vi "获取队列引用.vi"(8 "错误输入（无错误）":errorcluster) -> (0 "错误输出":errorcluster, 3 "队列组":T1)   [LabVIEW 2020]
uses:
  viLib/QueueLib/QueueLib.lvlib
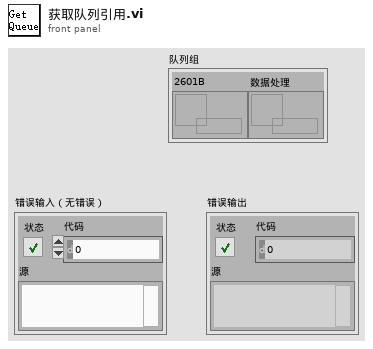
[diagram p1: front panel]
types:
  T1 = typedef "队列组.ctl" = cluster{"2601B":refnum<queue>, "数据处理":refnum<queue>}
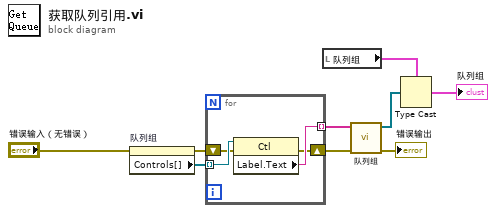
[diagram p0: block diagram]
diagram:
  n1 = property on="队列组" class="Clust (严格)"(error in="错误输入（无错误）") -> (error out=w3:errorcluster, "Controls[]"=w6:refnum<vi>[])  [unwired: 1 in, 1 out]
  n2 = for {
    tunnel: w6 -> [w13] mode=indexing
    tunnel: [w12] -> w5 mode=indexing
    shift-right: [w10] -> w2
    shift-left: w3 -> [w11]
    n3 = property class="Ctl"(reference=w13, error in=w11) -> (error out=w10:errorcluster, "Label.Text"=w12:string)  [unwired: 1 out]
  }
  n4 = local read "队列组"() -> (w1:T1)
  n5 = call "队列组.vi"("错误输入（无错误）"=w2, "队列名称"=w5) -> ("错误输出"=→"错误输出":errorcluster, "队列组"=w8:refnum<queue>[])  [unwired: 8 in]
  n6 = Type Cast(type=w1, x=w8) -> (*(type *) &x=→"队列组":T1)
